vi "Initialize.vi"(8 "error in":errorcluster, 9 "Slot Settings":T1, 11 "9216 in":refnum<class "9216.lvclass">) -> (0 "error out":errorcluster, 3 "9216 out":refnum<class "9216.lvclass">)   [LabVIEW 2017, in "Modules.lvlib" / "9216.lvclass"]
uses:
  9216.lvclass
  C:/Users/nitest/Documents/NI/niveristand-scan-engine-module-libraries/Source/RSI Module/RSI Module.lvclass
  RSI Module/Slot Settings.ctl
  RSI Module/Channels.ctl
  RSI Module/Channel Type.ctl
  RSI Module/Module Models.ctl
  9216.lvclass/9216.ctl
  RSI Module/RSI Module.lvclass
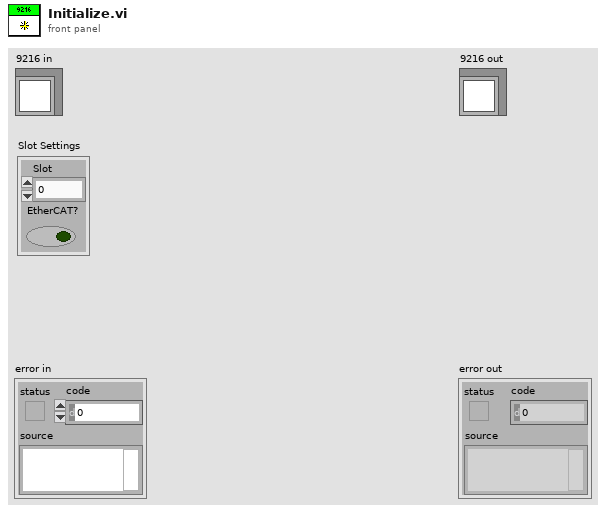
[diagram p1: front panel]
types:
  T1 = typedef "Modules.lvlib/RSI Module.lvclass/Slot Settings.ctl" = cluster{"Slot":u32, "EtherCAT?":bool}
  T2 = typedef "Modules.lvlib/RSI Module.lvclass/Channels.ctl" = cluster{"# Input Channels":i32, "# Output Channels":i32, "Channel Type":T3, "Units":string}
  T3 = typedef "Modules.lvlib/RSI Module.lvclass/Channel Type.ctl" = enum16{"Analog", "Digital"}
  T4 = cluster{"Ohm degree range":u32, "RTD type":u32, "RTD user-defined A constant":dbl, "RTD user-defined B constant":dbl, "RTD user-defined C constant":dbl, "RTD user-defined Ro constant":dbl}
  T5 = typedef "Modules.lvlib/RSI Module.lvclass/Module Models.ctl" = enum16{"Empty", "NI 9201", "NI 9203", "NI 9205", "NI 9206", "NI 9207", "NI 9208", "NI 9209", "NI 9211", "NI 9212", "NI 9213", "NI 9214", "NI 9215", "NI 9216", "NI 9217", "NI 9219", "NI 9220", "NI 9221", "NI 9222", "NI 9223", "NI 9224", "NI 9225", "NI 9227", "NI 9228", "NI 9229", "NI 9233", "NI 9234", "NI 9235", "NI 9236", "NI 9237", "NI 9239", "NI 9242", "NI 9244", "NI 9263", "NI 9264", "NI 9265", "NI 9266", "NI 9269", "NI 9344", "NI 9350", "NI 9375", "NI 9401", "NI 9402", "NI 9403", "NI 9411", "NI 9421", "NI 9422", "NI 9423", "NI 9425", "NI 9426", "NI 9435", "NI 9436", "NI 9437", "NI 9472", "NI 9474", "NI 9475", "NI 9476", "NI 9477", "NI 9478", "NI 9481", "NI 9482", "NI 9485"}
  T6 = cluster{"Ohm degree range":u32, "RTD type":u32, "RTD user-defined A constant":dbl, "RTD user-defined B constant":dbl, "RTD user-defined C constant":dbl, "RTD user-defined Ro constant":dbl}[]
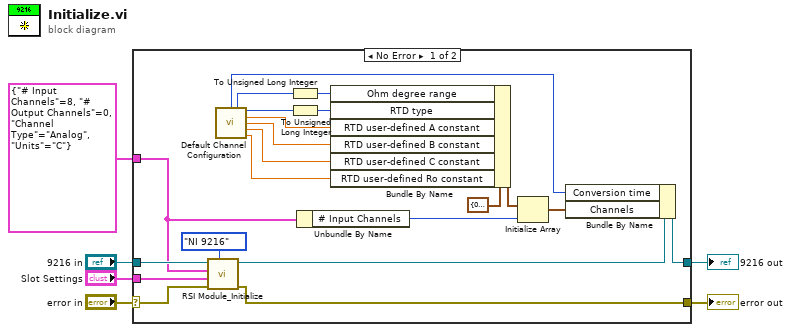
[diagram p0: block diagram]
diagram:
  n1 = case shown="No Error" "error in" {
    selector: "error in" -> [w26 w29]
    tunnel: [w25 w29] -> w3
    tunnel: [w17 w28] -> w5
    tunnel: "Slot Settings" -> [w27 _]
    tunnel: "9216 in" -> [w22 w28]
    tunnel: T2 {"# Input Channels"=8, "# Output Channels"=0, "Channel Type"=enum."Analog", "Units"="C"} ("Channels") -> [w16 _]
    frame No Error {
      n2 = call "RSI Module_Initialize.vi"("Module Model"=Module_Models."NI 9216", "error in (no error)"=w26, "Slot Settings"=w27, "Channels"=w16, "RSI Module in"=w22) -> ("error out"=w25:errorcluster, "RSI Module out"=w24:refnum<class "9216.lvclass">)  [unwired: 5 in]
      n3 = call "Default Channel Configuration.vi"() -> ("Conversion Time"=w15:u16, "Degree Range"=w14:u8, "RTD Types"=w13:u8, "RTD_A"=w12:dbl, "RTD_B"=w11:dbl, "RTD_C"=w10:dbl, "RTD_Ro"=w9:dbl)  [unwired: 9 in]
      n4 = To Unsigned Long Integer(number=w14) -> (unsigned 32bit integer=w8:u32)
      n5 = To Unsigned Long Integer(number=w13) -> (unsigned 32bit integer=w7:u32)
      n6 = Unbundle By Name(w16) -> ("# Input Channels"=w19:i32)
      n7 = Bundle By Name(cluster=T4 {"Ohm degree range"=0, "RTD type"=0, "RTD user-defined A constant"=0.0, "RTD user-defined B constant"=0.0, "RTD user-defined C constant"=0.0, "RTD user-defined Ro constant"=0.0} ("Channel"), "Ohm degree range"=w8, "RTD type"=w7, "RTD user-defined A constant"=w12, "RTD user-defined B constant"=w11, "RTD user-defined C constant"=w10, "RTD user-defined Ro constant"=w9) -> (w20:T4)
      n8 = Initialize Array(w20, w19) -> (w18:T6)
      n9 = Bundle By Name(cluster=w24, "Conversion time"=w15, "Channels"=w18) -> (w17:refnum<class "9216.lvclass">)
    }
    frame Error {
    }
  }
  "error out" <- w3
  "9216 out" <- w5
